vi "NET_Gear.vi"(8 "Read(F) Write(T)":bool, 11 "High Gear In":bool) -> (3 "High Gear Out":bool)   [LabVIEW 2017]
uses:
  <vilib>/Rock Robotics/Network Tables/NT Read Boolean.vi
  <vilib>/Rock Robotics/Network Tables/NT Write Boolean.vi
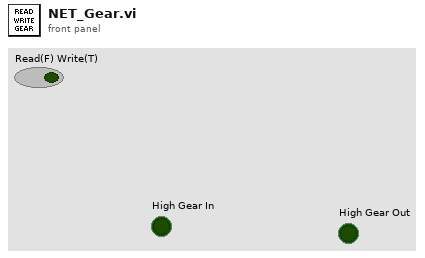
[diagram p1: front panel]
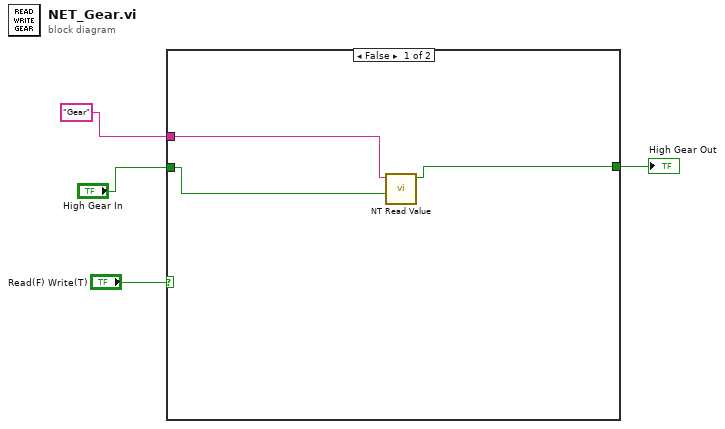
[diagram p0: block diagram]
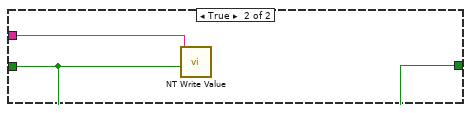
[diagram p2: hidden frame]
diagram:
  n1 = case shown="False" "Read(F) Write(T)" {
    tunnel: "Gear" ("Name") -> [w7 w9]
    tunnel: "High Gear In" -> [w6 w8]
    tunnel: [w5 w8] -> w1
    frame False {
      n2 = call-poly <vilib>:"NT Read Value.vi"("Default Value"=w6, "Name"=w7) -> ("Boolean"=w5:bool)  [unwired: 8 in, 1 out]
    }
    frame True {
      n3 = call-poly <vilib>:"NT Write Value.vi"("Boolean"=w8, "Name"=w9) -> ()  [unwired: 9 in, 1 out]
    }
  }
  "High Gear Out" <- w1
